vi "显示UI.vi"() -> ()   [LabVIEW 2016, in "国弘多参数.lvlib"]
uses:
  <vilib>/Utility/miscctls.llb/LVPointTypeDef.ctl
  <vilib>/Utility/config.llb/NI_LVConfig.lvlib
panel:
  in  "周期设置":bool
  out "运行状态":u16(ring) items=["空闲", "水样测试", "标样核查"]
  in  "叶绿素a校准":bool
  in  "停止":bool
  in  "标样核查":bool
  in  "水样测试":bool
  in  "open MB":bool
  in  "设置":bool
  in  "水温校准":bool
  in  "浊度校准":bool
  in  "溶解氧校准":bool
  in  "电导率校准":bool
  in  "pH校准":bool
  in  "探头校正返回":bool
  in  "探头校正":bool
  in  "浊度参数查询":bool
  in  "溶解氧参数查询":bool
  in  "电导率参数查询":bool
  in  "pH参数查询":bool
  out "检测值":T1
  in  "返回":bool
  in  "参数查询":bool
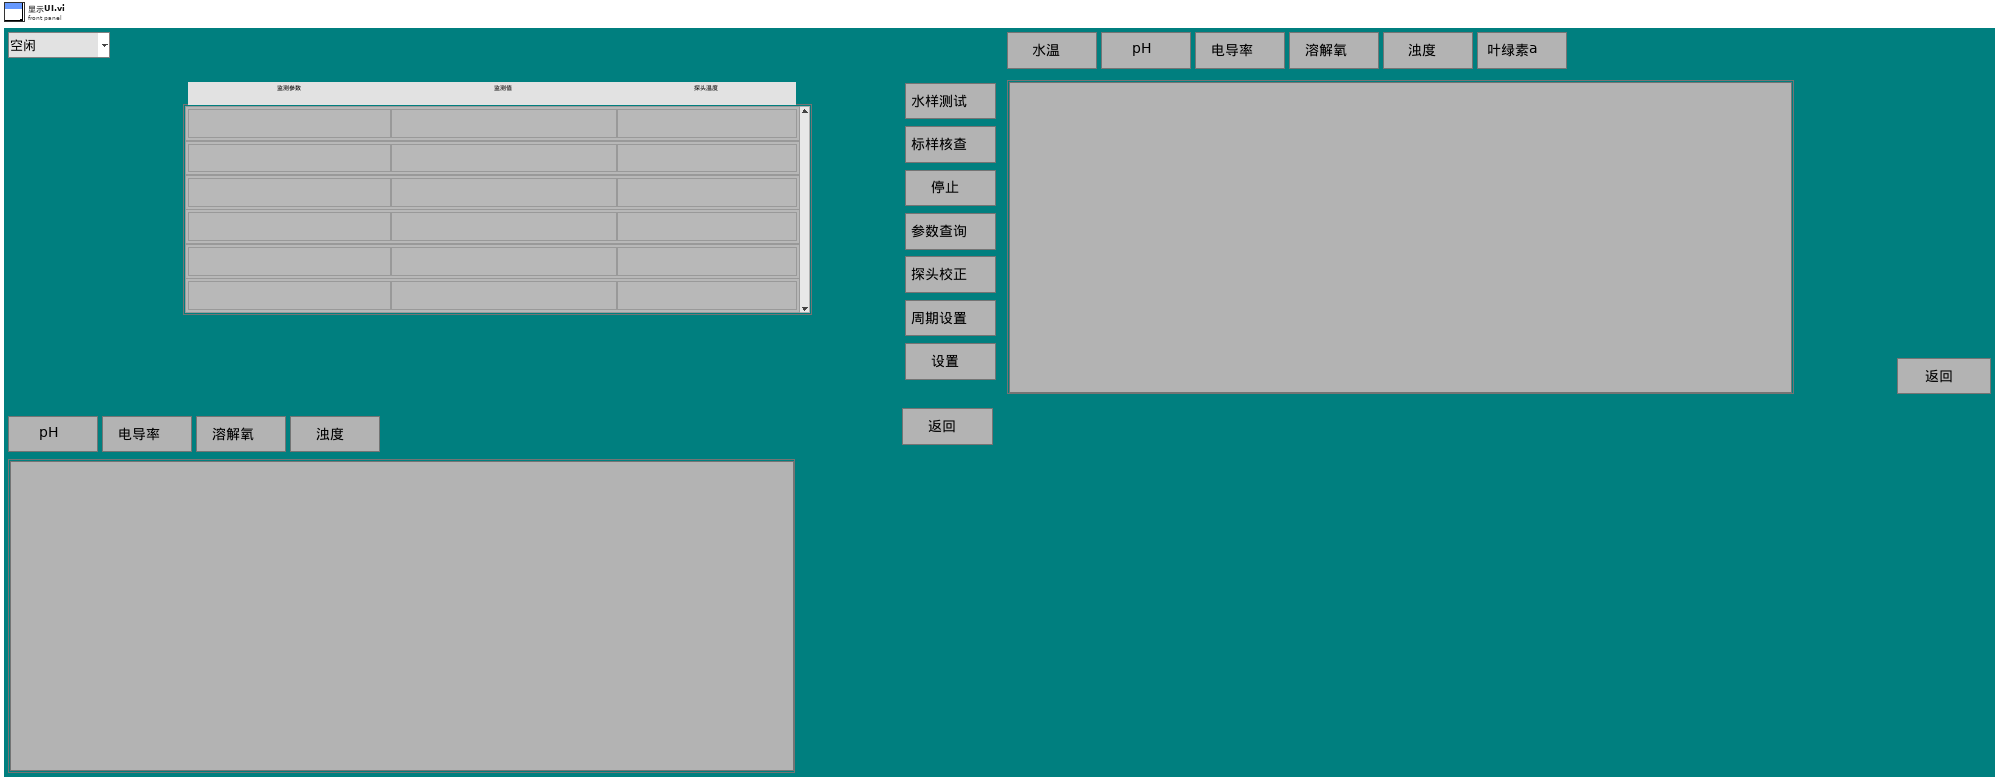
[diagram p1: front panel]
types:
  T1 = typedef "国弘多参数.lvlib/检测值.ctl" = cluster{"监测参数1":string, "浓度1":string, "探头温度1":string}[]
  T2 = typedef "LVPointTypeDef.ctl" = cluster{"Horizontal":i16, "Vertical":i16}
  T3 = cluster{"电极状态标志":u16, "电极型号标志":u16, "溶解氧测量值":sgl, "温度测量值":sgl, "溶解氧饱和度值":sgl, "盐度补偿值":sgl, "大气压补偿值":sgl, "溶解氧偏移修正值":sgl, "温度偏移修正值":sgl, "手动温度补偿值":sgl, "溶解氧电极零点":sgl, "溶解氧电极斜率":sgl, "第1点标准值记录":sgl, "第1点信号值记录":sgl, "第1点温度值记录":sgl, "第2点标准值记录":sgl, "第2点信号值记录":sgl, "第2点温度值记录":sgl, "命令滤波设定":u16, "温度模式":enum16{"ATC", "MTC"}, "生产批次":u16, "电极序号":u16, "串口地址":u16, "串口波特率":enum16{"9600", "19200", "115200"}, "串口校验位":enum16{"NONE", "ODD", "EVEN"}, "串口停止位":enum16{"1bit", "2bit"}, "第一点标准值":sgl, "第二点标准值":sgl}
  T4 = cluster{"电极状态标志":u16, "电极型号标志":u16, "酸碱度测量值":sgl, "温度测量值":sgl, "酸碱度信号值":sgl, "温度信号值":sgl, "酸碱度偏移修正值":sgl, "温度偏移修正值":sgl, "手动温度补偿值":sgl, "酸碱度电极零点":sgl, "酸碱度电极斜率":sgl, "第1点标准值记录":sgl, "第1点信号值记录":sgl, "第1点温度值记录":sgl, "第2点标准值记录":sgl, "第2点信号值记录":sgl, "第2点温度值记录":sgl, "命令滤波设定":u16, "温度模式":enum16{"ATC", "MTC"}, "生产批次":u16, "电极序号":u16, "串口地址":u16, "串口波特率":enum16{"9600", "19200", "115200"}, "串口校验位":enum16{"NONE", "ODD", "EVEN"}, "串口停止位":enum16{"1bit", "2bit"}, "第一点标准值":sgl, "第二点标准值":sgl}
  T5 = cluster{"电极状态标志":u16, "电极型号标志":u16, "浊度测量值":sgl, "温度测量值":sgl, "浊度信号值":sgl, "浊度偏移修正值":sgl, "温度偏移修正值":sgl, "手动温度补偿值":sgl, "浊度电极零点":sgl, "浊度电极斜率":sgl, "第1点标准值记录":sgl, "第1点信号值记录":sgl, "第1点温度值记录":sgl, "第2点标准值记录":sgl, "第2点信号值记录":sgl, "第2点温度值记录":sgl, "命令滤波设定":u16, "温度模式":enum16{"ATC", "MTC"}, "生产批次":u16, "电极序号":u16, "串口地址":u16, "串口波特率":enum16{"9600", "19200", "115200"}, "串口校验位":enum16{"NONE", "ODD", "EVEN"}, "串口停止位":enum16{"1bit", "2bit"}, "第一点标准值":sgl, "第二点标准值":sgl}
  T6 = cluster{"电极状态标志":u16, "电极型号标志":u16, "电导率测量值":sgl, "温度测量值":sgl, "电导率信号值":sgl, "温度信号值":sgl, "温度补偿系数":sgl, "电导率偏移修正值":sgl, "温度偏移修正值":sgl, "手动温度补偿值":sgl, "电导率电极零点":sgl, "电导率电极斜率":sgl, "命令滤波设定":u16, "温度模式":enum16{"ATC", "MTC"}, "生产批次":u16, "电极序号":u16, "串口地址":u16, "串口波特率":enum16{"9600", "19200", "115200"}, "串口校验位":enum16{"NONE", "ODD", "EVEN"}, "串口停止位":enum16{"1bit", "2bit"}, "第一点标准值":sgl, "第二点标准值":sgl}
  T7 = cluster{"监测参数1":string, "浓度1":string, "探头温度1":string}[]
  T8 = cluster{"CH":u16, "监测值":dbl, "监测信号值":dbl, "温度偏移修正值":sgl}
  T9 = typedef "NI_LVConfig.lvlib/Config Data RefNum.ctl" = refnum<k1>
  T10 = enum32{"Bad", "Idle", "Run top level", "Running"}
  T11 = cluster{"baud rate (bps)":u32, "stop bits":u16, "parity":u16, "flow control":u16, "timeout":u32, "retries":i32}
  T12 = enum32{"Invalid", "Standard", "Closed", "Hidden", "Minimized", "Maximized"}
  T13 = cluster{"数据保存间隔":dbl, "水温标样值":dbl, "pH标样值":dbl, "溶解氧标样值":dbl, "电导率标样值":dbl, "浊度标样值":dbl}
  T14 = cluster{"Temp":bool, "pH":bool, "DO":bool, "Cond":bool, "Turb":bool, "叶绿素a启用":bool}
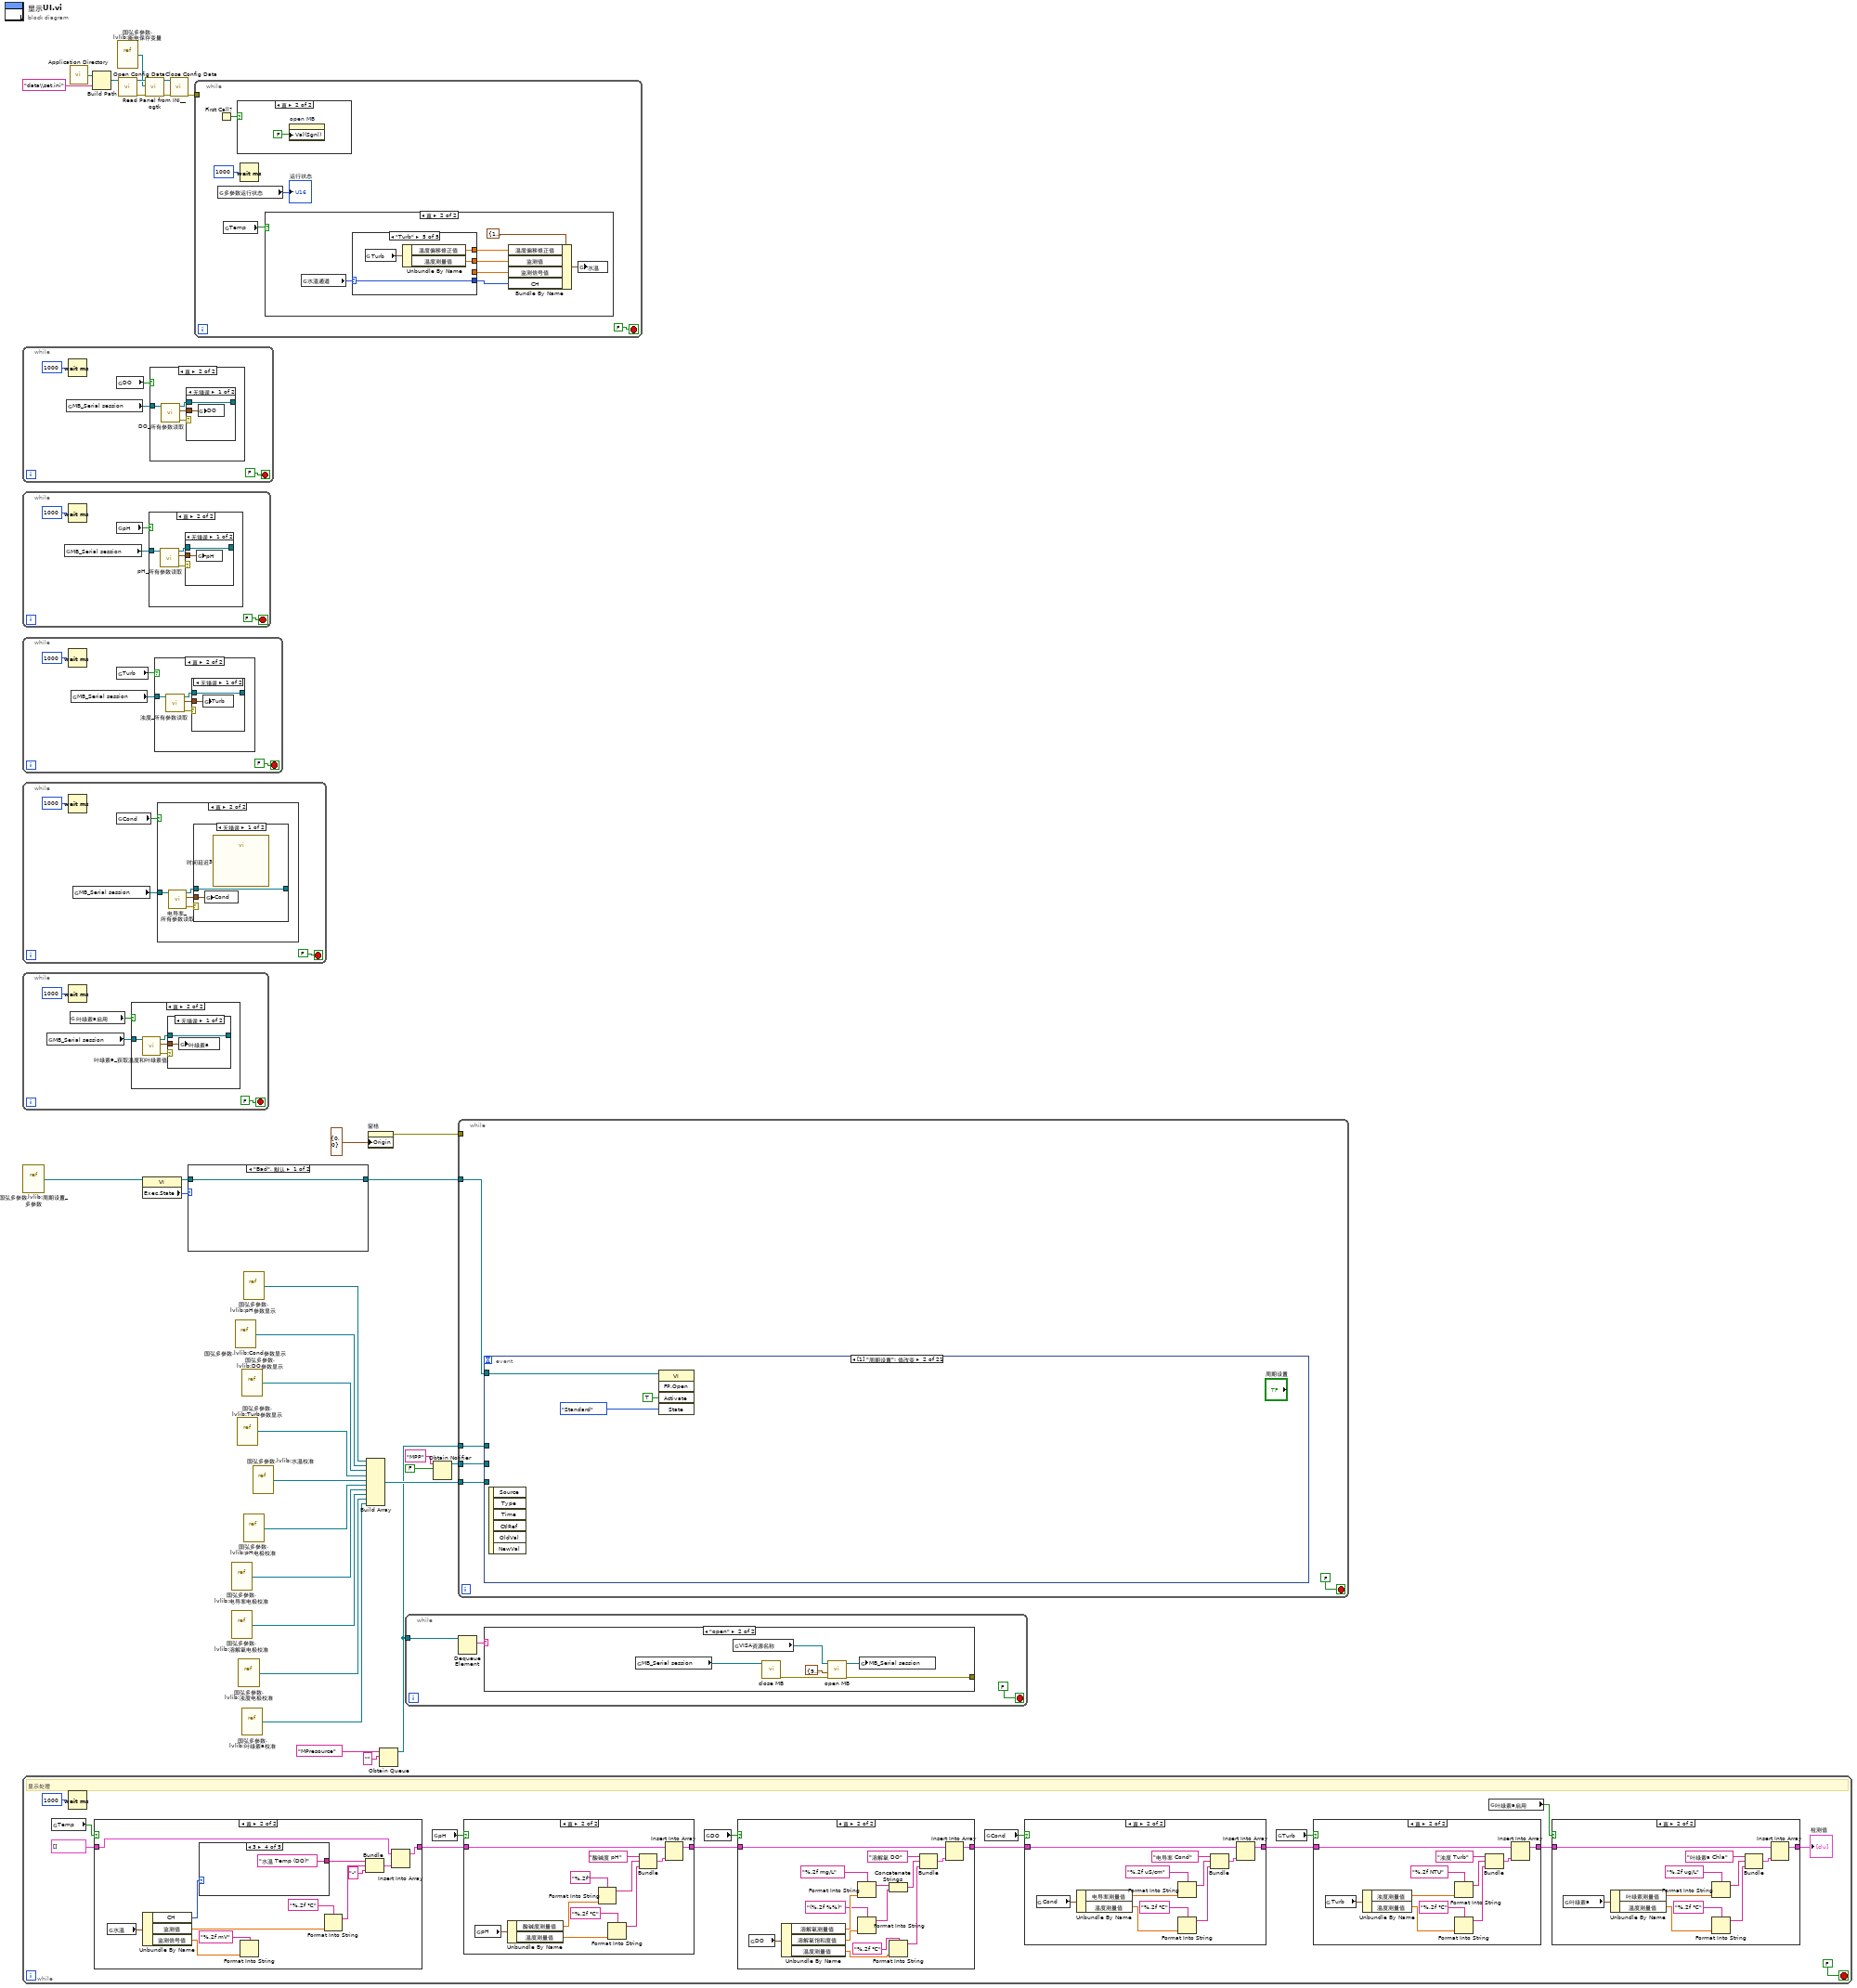
[diagram p0: block diagram]
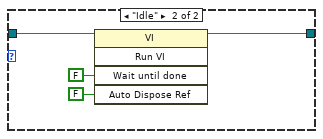
[diagram p2: hidden frame]
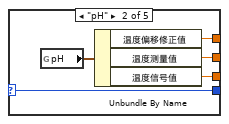
[diagram p16: hidden frame]
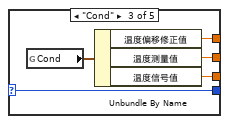
[diagram p17: hidden frame]
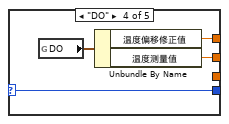
[diagram p18: hidden frame]
diagram:
  n1 = while {
    stop <- FALSE stop-if-true
    n2 = global read "过程全局变量.vi" "MB_Serial session"() -> (w33:refnum<class "MB_Master_Serial.lvclass">)
    n3 = Wait (ms)(milliseconds to wait=u32 1000 ("等待时间（毫秒）")) -> ()  [unwired: 1 out]
    n4 = global read "断电保存变量.vi" "DO"() -> (w34:bool)
    n5 = case shown="真" w34 {
      tunnel: w33 -> [_ w37]
      frame False {
      }
      frame True {
        n6 = call "DO_所有参数读取.vi"("MB_Serial session in"=w37) -> ("error out"=w39:errorcluster, "输出值"=w40:T3, "MB_Serial session out"=w38:refnum<class "MB_Master_Serial.lvclass">)  [unwired: 8 in]
        n7 = case shown="无错误" w39 {
          tunnel: w40 -> [w42 _]
          tunnel: w38 -> [w41 w43]
          tunnel: [w41 w43] -> _
          frame No Error {
            n8 = global write "过程全局变量.vi" "DO"(w42) -> ()
          }
          frame Error {
          }
        }
      }
    }
  }
  n9 = while {
    stop <- FALSE stop-if-true
    n10 = global read "过程全局变量.vi" "MB_Serial session"() -> (w45:refnum<class "MB_Master_Serial.lvclass">)
    n11 = Wait (ms)(milliseconds to wait=u32 1000 ("等待时间（毫秒）")) -> ()  [unwired: 1 out]
    n12 = global read "断电保存变量.vi" "pH"() -> (w46:bool)
    n13 = case shown="真" w46 {
      tunnel: w45 -> [_ w48]
      frame False {
      }
      frame True {
        n14 = call "pH_所有参数读取.vi"("MB_Serial session in"=w48) -> ("error out"=w50:errorcluster, "输出值"=w51:T4, "MB_Serial session out"=w49:refnum<class "MB_Master_Serial.lvclass">)  [unwired: 8 in]
        n15 = case shown="无错误" w50 {
          tunnel: w51 -> [w53 _]
          tunnel: w49 -> [w52 w54]
          tunnel: [w52 w54] -> _
          frame No Error {
            n16 = global write "过程全局变量.vi" "pH"(w53) -> ()
          }
          frame Error {
          }
        }
      }
    }
  }
  n17 = while {
    stop <- FALSE stop-if-true
    n18 = Wait (ms)(milliseconds to wait=u32 1000 ("等待时间（毫秒）")) -> ()  [unwired: 1 out]
    n19 = global read "过程全局变量.vi" "MB_Serial session"() -> (w56:refnum<class "MB_Master_Serial.lvclass">)
    n20 = global read "断电保存变量.vi" "Turb"() -> (w57:bool)
    n21 = case shown="真" w57 {
      tunnel: w56 -> [_ w59]
      frame False {
      }
      frame True {
        n22 = call "浊度_所有参数读取.vi"("MB_Serial session in"=w59) -> ("error out"=w61:errorcluster, "输出值"=w62:T5, "MB_Serial session out"=w60:refnum<class "MB_Master_Serial.lvclass">)  [unwired: 8 in]
        n23 = case shown="无错误" w61 {
          tunnel: w62 -> [w64 _]
          tunnel: w60 -> [w63 w65]
          tunnel: [w63 w65] -> _
          frame No Error {
            n24 = global write "过程全局变量.vi" "Turb"(w64) -> ()
          }
          frame Error {
          }
        }
      }
    }
  }
  n25 = while {
    stop <- FALSE stop-if-true
    n26 = Wait (ms)(milliseconds to wait=u32 1000 ("等待时间（毫秒）")) -> ()  [unwired: 1 out]
    n27 = global read "过程全局变量.vi" "MB_Serial session"() -> (w67:refnum<class "MB_Master_Serial.lvclass">)
    n28 = global read "断电保存变量.vi" "Cond"() -> (w68:bool)
    n29 = case shown="真" w68 {
      tunnel: w67 -> [_ w70]
      frame False {
      }
      frame True {
        n30 = call "电导率_所有参数读取.vi"("MB_Serial session in"=w70) -> ("error out"=w72:errorcluster, "输出值"=w73:T6, "MB_Serial session out"=w71:refnum<class "MB_Master_Serial.lvclass">)  [unwired: 8 in]
        n31 = case shown="无错误" w72 {
          tunnel: w73 -> [w75 _]
          tunnel: [w74 w76] -> _
          tunnel: w71 -> [w74 w76]
          frame No Error {
            n32 = global write "过程全局变量.vi" "Cond"(w75) -> ()
            n33 = call "时间延迟3"() -> ()  [unwired: 11 in, 1 out]
          }
          frame Error {
          }
        }
      }
    }
  }
  n34 = while {
    stop <- FALSE stop-if-true
    n35 = global read "过程全局变量.vi" "MB_Serial session"() -> (w79:refnum<class "MB_Master_Serial.lvclass">)
    n36 = Wait (ms)(milliseconds to wait=u32 1000 ("等待时间（毫秒）")) -> ()  [unwired: 1 out]
    n37 = global read "断电保存变量.vi" "叶绿素a启用"() -> (w78:bool)
    n38 = case shown="真" w78 {
      tunnel: w79 -> [_ w81]
      frame False {
      }
      frame True {
        n39 = call "叶绿素a_获取温度和叶绿素值.vi"("MB_Serial session in"=w81) -> ("error out"=w83:errorcluster, "输出值"=w84:cluster{"温度测量值":sgl, "叶绿素测量值":sgl, "错误标志":u16}, "MB_Serial session out"=w82:refnum<class "MB_Master_Serial.lvclass">)  [unwired: 8 in]
        n40 = case shown="无错误" w83 {
          tunnel: w84 -> [w86 _]
          tunnel: w82 -> [w85 w87]
          tunnel: [w85 w87] -> _
          frame No Error {
            n41 = global write "过程全局变量.vi" "叶绿素a"(w86) -> ()
          }
          frame Error {
          }
        }
      }
    }
  }
  n42 = vi-ref "国弘多参数.lvlib:周期设置_多参数.vi"() -> (w4:refnum<vi>)
  n43 = while {
    stop <- FALSE stop-if-true
    # "显示处理"
    n44 = global read "断电保存变量.vi" "Temp"() -> (w100:bool)
    n45 = Wait (ms)(milliseconds to wait=u32 1000 ("等待时间（毫秒）")) -> ()  [unwired: 1 out]
    n46 = case shown="真" w100 {
      tunnel: [w167 w168] -> w97
      tunnel: T7 [] ("数组") -> [w167 w169]
      frame False {
      }
      frame True {
        n47 = global read "过程全局变量.vi" "水温"() -> (w179:T8)
        n48 = Unbundle By Name(w179) -> ("CH"=w174:u16, "监测值"=w177:dbl, "监测信号值"=w175:dbl)
        n49 = case shown="3" w174 {
          tunnel: ["水温 Temp" ("监测参数1") "水温 Temp (pH)" ("监测参数1") "水温 Temp (Cond)" ("监测参数1") "水温 Temp (DO)" ("监测参数1") "水温 Temp (Turb)" ("监测参数1")] -> w173
          frame 0, Default {
          }
          frame 1 {
          }
          frame 2 {
          }
          frame 3 {
          }
          frame 4 {
          }
        }
        n50 = Format Into String(format string="%.2f mV" ("格式字符串"), w175) -> ()  [unwired: 2 in, 2 out]
        n51 = Format Into String(format string="%.2f ℃" ("格式字符串"), w177) -> (resulting string=w172:string)  [unwired: 2 in, 1 out]
        n52 = Bundle("监测参数1"=w173, w172, "探头温度1"="-") -> (w170:cluster{"监测参数1":string, string, "探头温度1":string})  [unwired: 1 in]
        n53 = Insert Into Array(array=w169, new element=w170) -> (w168:T7)  [unwired: 1 in]
      }
    }
    n54 = global read "断电保存变量.vi" "pH"() -> (w98:bool)
    n55 = case shown="真" w98 {
      tunnel: [w155 w156] -> w95
      tunnel: w97 -> [w155 w158]
      frame False {
      }
      frame True {
        n56 = global read "过程全局变量.vi" "pH"() -> (w166:T4)
        n57 = Unbundle By Name(w166) -> ("酸碱度测量值"=w165:sgl, "温度测量值"=w163:sgl)
        n58 = Format Into String(format string="%.2f" ("格式字符串"), w165) -> (resulting string=w159:string)  [unwired: 2 in, 1 out]
        n59 = Format Into String(format string="%.2f ℃" ("格式字符串"), w163) -> (resulting string=w161:string)  [unwired: 2 in, 1 out]
        n60 = Bundle("监测参数2"="酸碱度 pH", w159, w161) -> (w157:cluster{"监测参数2":string, string, string})  [unwired: 1 in]
        n61 = Insert Into Array(array=w158, new element=w157) -> (w156:T7)  [unwired: 1 in]
      }
    }
    n62 = global read "断电保存变量.vi" "DO"() -> (w96:bool)
    n63 = case shown="真" w96 {
      tunnel: [w139 w140] -> w92
      tunnel: w95 -> [w139 w141]
      frame False {
      }
      frame True {
        n64 = global read "过程全局变量.vi" "DO"() -> (w150:T3)
        n65 = Unbundle By Name(w150) -> ("溶解氧测量值"=w151:sgl, "溶解氧饱和度值"=w148:sgl, "温度测量值"=w153:sgl)
        n66 = Format Into String(format string="%.2f mg/L" ("格式字符串"), w151) -> (resulting string=w147:string)  [unwired: 2 in, 1 out]
        n67 = Format Into String(format string="(%.2f %%)" ("格式字符串"), w148) -> (resulting string=w146:string)  [unwired: 2 in, 1 out]
        n68 = Concatenate Strings(w147, w146) -> (w145:string)
        n69 = Format Into String(format string="%.2f ℃" ("格式字符串"), w153) -> (resulting string=w143:string)  [unwired: 2 in, 1 out]
        n70 = Bundle("监测参数2"="溶解氧 DO", w145, w143) -> (w142:cluster{"监测参数2":string, string, string})  [unwired: 1 in]
        n71 = Insert Into Array(array=w141, new element=w142) -> (w140:T7)  [unwired: 1 in]
      }
    }
    n72 = global read "断电保存变量.vi" "Cond"() -> (w94:bool)
    n73 = case shown="真" w94 {
      tunnel: w92 -> [w127 w130]
      tunnel: [w127 w128] -> w91
      frame False {
      }
      frame True {
        n74 = global read "过程全局变量.vi" "Cond"() -> (w138:T6)
        n75 = Unbundle By Name(w138) -> ("电导率测量值"=w137:sgl, "温度测量值"=w135:sgl)
        n76 = Format Into String(format string="%.2f uS/cm" ("格式字符串"), w137) -> (resulting string=w131:string)  [unwired: 2 in, 1 out]
        n77 = Format Into String(format string="%.2f ℃" ("格式字符串"), w135) -> (resulting string=w132:string)  [unwired: 2 in, 1 out]
        n78 = Bundle("监测参数2"="电导率 Cond", w131, w132) -> (w129:cluster{"监测参数2":string, string, string})  [unwired: 1 in]
        n79 = Insert Into Array(array=w130, new element=w129) -> (w128:T7)  [unwired: 1 in]
      }
    }
    n80 = global read "断电保存变量.vi" "Turb"() -> (w93:bool)
    n81 = case shown="真" w93 {
      tunnel: w91 -> [w115 w118]
      tunnel: [w115 w116] -> w90
      frame False {
      }
      frame True {
        n82 = global read "过程全局变量.vi" "Turb"() -> (w122:T5)
        n83 = Unbundle By Name(w122) -> ("浊度测量值"=w123:sgl, "温度测量值"=w125:sgl)
        n84 = Format Into String(format string="%.2f NTU" ("格式字符串"), w123) -> (resulting string=w120:string)  [unwired: 2 in, 1 out]
        n85 = Format Into String(format string="%.2f ℃" ("格式字符串"), w125) -> (resulting string=w121:string)  [unwired: 2 in, 1 out]
        n86 = Bundle("监测参数2"="浊度 Turb", w120, w121) -> (w117:cluster{"监测参数2":string, string, string})  [unwired: 1 in]
        n87 = Insert Into Array(array=w118, new element=w117) -> (w116:T7)  [unwired: 1 in]
      }
    }
    n88 = global read "断电保存变量.vi" "叶绿素a启用"() -> (w88:bool)
    n89 = case shown="真" w88 {
      tunnel: w90 -> [w103 w106]
      tunnel: [w103 w104] -> w89
      frame False {
      }
      frame True {
        n90 = global read "过程全局变量.vi" "叶绿素a"() -> (w110:cluster{"温度测量值":sgl, "叶绿素测量值":sgl, "错误标志":u16})
        n91 = Unbundle By Name(w110) -> ("叶绿素测量值"=w111:sgl, "温度测量值"=w113:sgl)
        n92 = Format Into String(format string="%.2f ug/L" ("格式字符串"), w111) -> (resulting string=w108:string)  [unwired: 2 in, 1 out]
        n93 = Format Into String(format string="%.2f ℃" ("格式字符串"), w113) -> (resulting string=w109:string)  [unwired: 2 in, 1 out]
        n94 = Bundle("监测参数2"="叶绿素a Chla", w108, w109) -> (w105:cluster{"监测参数2":string, string, string})  [unwired: 1 in]
        n95 = Insert Into Array(array=w106, new element=w105) -> (w104:T7)  [unwired: 1 in]
      }
    }
    "检测值" <- w89
  }
  n96 = call <vilib>:"Application Directory.vi"() -> ("Application Directory"=w16:path)
  n97 = Build Path(base path=w16, name or relative path="data\\set.ini" ("名称或相对路径")) -> (appended path=w15:path)
  n98 = vi-ref "国弘多参数.lvlib:断电保存变量.vi"() -> (w13:refnum<vi>)
  n99 = call <vilib>:"Open Config Data.vi"("configuration file path"=w15) -> ("error out"=w19:errorcluster, "refnum"=w20:T9)  [unwired: 8 in, 1 out]
  n100 = property class="VI"(reference=w4) -> (reference out=w2:refnum<vi>, "Exec.State"=w3:T10)  [unwired: 1 in, 1 out]
  n101 = call <userlib>:"Read Panel from INI__ogtk.vi"("error in (no error)"=w19, "VI ref"=w13, "refnum"=w20) -> ("error out"=w17:errorcluster, "refnum out"=w18:T9)  [unwired: 7 in]
  n102 = call <vilib>:"Close Config Data.vi"("error in (no error)"=w17, "refnum"=w18) -> ("error out"=w12:errorcluster)  [unwired: 8 in, 1 out]
  n103 = case shown="\"Bad\", 默认" w3 {
    tunnel: w2 -> [w185 w189]
    tunnel: [w185 w186] -> w1
    frame "Bad", Default {
    }
    frame "Idle" {
      n104 = invoke class="VI" method="Run VI"(reference=w189, "Wait until done"=FALSE ("结束前等待"), "Auto Dispose Ref"=FALSE ("自动销毁引用")) -> (reference out=w186:refnum<vi>)  [unwired: 2 in, 4 out]
    }
  }
  n105 = while {
    tunnel: w12 -> [_]
    stop <- FALSE stop-if-true
    n106 = First Call?() -> (First Call?: T/F=w192:bool)
    n107 = global read "过程全局变量.vi" "多参数运行状态"() -> (→"运行状态":u16)
    n108 = global read "断电保存变量.vi" "Temp"() -> (w191:bool)
    n109 = case shown="真" w192 {
      frame False {
      }
      frame True {
        n110 = property on="open MB" class="Bool (严格)"("Val(Sgnl)"=FALSE ("值(信号)")) -> ()  [unwired: 2 in, 2 out]
      }
    }
    n111 = Wait (ms)(milliseconds to wait=u32 1000 ("等待时间（毫秒）")) -> ()  [unwired: 1 out]
    n112 = case shown="真" w191 {
      frame False {
      }
      frame True {
        n113 = global read "断电保存变量.vi" "水温通道"() -> (w201:enum16{"NULL", "pH", "Cond", "DO", "Turb"})
        n114 = case shown="\"Turb\"" w201 {
          selector: w201 -> [w202 w207 w212 w216 w220]
          tunnel: [w202 w207 w212 w216 w220] -> w200
          tunnel: [_ w205 w210 w214 w218] -> w199
          tunnel: [_ w204 w209 _ _] -> w198
          tunnel: [_ w203 w208 w213 w217] -> w195
          frame "NULL", Default {
          }
          frame "pH" {
            n115 = global read "过程全局变量.vi" "pH"() -> (w206:T4)
            n116 = Unbundle By Name(w206) -> ("温度偏移修正值"=w203:sgl, "温度测量值"=w205:sgl, "温度信号值"=w204:sgl)
          }
          frame "Cond" {
            n117 = global read "过程全局变量.vi" "Cond"() -> (w211:T6)
            n118 = Unbundle By Name(w211) -> ("温度偏移修正值"=w208:sgl, "温度测量值"=w210:sgl, "温度信号值"=w209:sgl)
          }
          frame "DO" {
            n119 = global read "过程全局变量.vi" "DO"() -> (w215:T3)
            n120 = Unbundle By Name(w215) -> ("温度偏移修正值"=w213:sgl, "温度测量值"=w214:sgl)
          }
          frame "Turb" {
            n121 = global read "过程全局变量.vi" "Turb"() -> (w219:T5)
            n122 = Unbundle By Name(w219) -> ("温度偏移修正值"=w217:sgl, "温度测量值"=w218:sgl)
          }
        }
        n123 = Bundle By Name(cluster=T8 {"CH"=1, "监测值"=0.0, "监测信号值"=0.0, "温度偏移修正值"=0.0} ("水温"), "温度偏移修正值"=w195, "监测值"=w199, "监测信号值"=w198, "CH"=w200) -> (w197:T8)
        n124 = global write "过程全局变量.vi" "水温"(w197) -> ()
      }
    }
  }
  n125 = vi-ref "国弘多参数.lvlib:电导率电极校准.vi"() -> (w23:refnum<vi>)
  n126 = vi-ref "国弘多参数.lvlib:溶解氧电极校准.vi"() -> (w22:refnum<vi>)
  n127 = vi-ref "国弘多参数.lvlib:Cond参数显示.vi"() -> (w29:refnum<vi>)
  n128 = vi-ref "国弘多参数.lvlib:Turb参数显示.vi"() -> (w27:refnum<vi>)
  n129 = vi-ref "国弘多参数.lvlib:浊度电极校准.vi"() -> (w21:refnum<vi>)
  n130 = vi-ref "国弘多参数.lvlib:DO参数显示.vi"() -> (w28:refnum<vi>)
  n131 = vi-ref "国弘多参数.lvlib:叶绿素a校准.vi"() -> (w11:refnum<vi>)
  n132 = vi-ref "国弘多参数.lvlib:pH参数显示.vi"() -> (w30:refnum<vi>)
  n133 = vi-ref "国弘多参数.lvlib:pH电极校准.vi"() -> (w24:refnum<vi>)
  n134 = vi-ref "国弘多参数.lvlib:水温校准.vi"() -> (w25:refnum<vi>)
  n135 = Build Array(w30, w29, w28, w27, w25, w24, w23, w22, w21, w11) -> (w26:refnum<vi>[])
  n136 = property on="窗格" class="Pane"("Origin"=T2 {"Horizontal"=0, "Vertical"=0} ("原点")) -> (error out=w32:errorcluster)  [unwired: 2 in, 1 out]
  n137 = Obtain Queue(name (unnamed)="MPresource" ("名称（未命名）"), element data type="" ("名称（未命名）")) -> (queue out=w5:refnum<queue>)  [unwired: 3 in, 2 out]
  n138 = while {
    tunnel: w5 -> [w223]
    stop <- FALSE stop-if-true
    n139 = Dequeue Element(queue=w223) -> (element=w222:string)  [unwired: 2 in, 3 out]
    n140 = case shown="\"open\"" w222 {
      tunnel: [_ w225] -> _
      frame "假", Default {
      }
      frame "open" {
        n141 = global read "过程全局变量.vi" "MB_Serial session"() -> (w230:refnum<class "MB_Master_Serial.lvclass">)
        n142 = global read "断电保存变量.vi" "VISA资源名称"() -> (w227:refnum<visa-resource-name>)
        n143 = call "close MB.vi"("MB_Serial session"=w230) -> ("error out"=w229:errorcluster)  [unwired: 10 in]
        n144 = call "open MB.vi"("error in (no error)"=w229, "Serial Config"=T11 {"baud rate (bps)"=9600, "stop bits"=10, "parity"=0, "flow control"=0, "timeout"=1000, "retries"=1}, "VISA资源名称"=w227) -> ("error out"=w225:errorcluster, "MB_Serial session"=w228:refnum<class "MB_Master_Serial.lvclass">)  [unwired: 7 in]
        n145 = global write "过程全局变量.vi" "MB_Serial session"(w228) -> ()
      }
    }
  }
  n146 = Obtain Notifier(name (unnamed)="MPP" ("名称（未命名）"), notification data type=FALSE) -> (notifier out=w8:refnum<notifier>)  [unwired: 2 in, 2 out]
  n147 = while {
    tunnel: w32 -> [_]
    tunnel: w26 -> [w234]
    tunnel: w8 -> [w233]
    tunnel: w5 -> [w232]
    tunnel: w1 -> [w231]
    stop <- FALSE stop-if-true
    n148 = event shown="[1] \"周期设置\": 值改变" {
      selector: _ -> [_ _ _ _ _ _ _ _ _ _ _ _ _ _ _ _ _ _ _ _ _]
      dyn-events: _ -> [_ _ _ _ _ _ _ _ _ _ _ _ _ _ _ _ _ _ _ _ _]
      timeout: _ -> [_ _ _ _ _ _ _ _ _ _ _ _ _ _ _ _ _ _ _ _ _]
      tunnel: w234 -> [_ _ _ _ _ _ _ w297 w310 w322 w330 w342 w354 w366 w378 w390 w402 w414 w426 w438 w450]
      tunnel: w233 -> [_ _ _ _ w270 _ _ _ _ _ _ _ _ _ _ _ _ _ _ _ _]
      tunnel: w232 -> [_ _ _ _ _ w273 _ _ _ _ _ _ _ _ _ _ _ _ _ _ _]
      tunnel: w231 -> [_ w238 _ _ _ _ _ _ _ _ _ _ _ _ _ _ _ _ _ _ _]
      event Timeout {
        n149 = event-data() -> ()  [unwired: 1 in, 3 out]
      }
      event "周期设置": Value Change {
        n150 = event-data() -> ()  [unwired: 1 in, 6 out]
        n151 = invoke class="VI" method="FP.Open"(reference=w238, "Activate"=TRUE ("激活？"), "State"=T12."Standard" ("状态")) -> ()  [unwired: 2 in, 5 out]
      }
      event "水样测试": Value Change {
        n152 = event-data() -> ()  [unwired: 1 in, 6 out]
        n153 = call "水样测试配置.vi"() -> ("确认输出"=w240:bool, "水样测定时间输出"=w239:dbl)  [unwired: 10 in]
        n154 = case shown="真" w240 {
          tunnel: w239 -> [_ w243]
          frame False {
          }
          frame True {
            n155 = vi-ref "国弘多参数.lvlib:水样测试.vi"() -> (w244:refnum<vi>)
            n156 = property class="VI"(reference=w244) -> ("Name"=w248:string, "Exec.State"=w246:T10)  [unwired: 1 in, 2 out]
            n157 = Open VI Reference(type specifier VI Refnum (for type only)=refnum<vi> refnum, vi path=w248, options=128 ("选项")) -> (vi reference=w249:refnum<vi>)  [unwired: 3 in, 1 out]
            n158 = case shown="\"Idle\"" w246 {
              tunnel: [w250 w254] -> w245
              tunnel: w249 -> [w250 w253]
              tunnel: w243 -> [_ w252]
              tunnel: "hd" ("数据标记表") -> [_ w251]
              frame "Bad", Default {
              }
              frame "Idle" {
                n159 = call-by-ref "开始异步调用"(reference=w253, "数据标记表"=w251, "水样测试时间"=w252) -> (reference out=w254:refnum<vi>)  [unwired: 11 in, 1 out]
              }
            }
            n160 = Close Reference(reference=w245) -> ()  [unwired: 1 in, 1 out]
          }
        }
      }
      event "标样核查": Value Change {
        n161 = event-data() -> ()  [unwired: 1 in, 6 out]
        n162 = call "标样核查配置.vi"() -> ("确认输出"=w256:bool, "标样核查配置"=w255:T13)  [unwired: 10 in]
        n163 = case shown="真" w256 {
          tunnel: w255 -> [_ w257]
          frame False {
          }
          frame True {
            n164 = vi-ref "国弘多参数.lvlib:标样核查.vi"() -> (w258:refnum<vi>)
            n165 = property class="VI"(reference=w258) -> ("Name"=w263:string, "Exec.State"=w260:T10)  [unwired: 1 in, 2 out]
            n166 = Open VI Reference(type specifier VI Refnum (for type only)=refnum<vi> refnum, vi path=w263, options=128 ("选项")) -> (vi reference=w264:refnum<vi>)  [unwired: 3 in, 1 out]
            n167 = case shown="\"Idle\"" w260 {
              tunnel: [w265 w268] -> w259
              tunnel: w264 -> [w265 w267]
              tunnel: w257 -> [_ w266]
              frame "Bad", Default {
              }
              frame "Idle" {
                n168 = call-by-ref "开始异步调用"(reference=w267, "标样核查配置"=w266) -> (reference out=w268:refnum<vi>)  [unwired: 12 in, 1 out]
              }
            }
            n169 = Close Reference(reference=w259) -> ()  [unwired: 1 in, 1 out]
          }
        }
      }
      event "停止": Value Change {
        n170 = event-data() -> ()  [unwired: 1 in, 6 out]
        n171 = Send Notification(notification=TRUE ("通知"), notifier=w270) -> ()  [unwired: 1 in, 2 out]
      }
      event "open MB": Value Change {
        n172 = event-data() -> ()  [unwired: 1 in, 6 out]
        n173 = Flush Queue(queue=w273) -> (queue out=w272:refnum<queue>)  [unwired: 1 in, 2 out]
        n174 = Enqueue Element(queue=w272, element="open" ("元素")) -> ()  [unwired: 2 in, 3 out]
      }
      event "设置": Value Change {
        n175 = event-data() -> ()  [unwired: 1 in, 6 out]
        n176 = flat-sequence {
          frame #0 {
            n177 = call "配置.vi"() -> ("启用参数"=w280:T14, "串口输出"=w281:refnum<visa-resource-name>)  [unwired: 10 in]
            n178 = global write "断电保存变量.vi" "VISA资源名称"(w281) -> ()
            n179 = Unbundle By Name(w280) -> ("Temp"=w275:bool, "pH"=w276:bool, "DO"=w277:bool, "Cond"=w278:bool, "Turb"=w279:bool, "叶绿素a启用"=w274:bool)
            n180 = global write "断电保存变量.vi" "pH"(w276) -> ()
            n181 = global write "断电保存变量.vi" "DO"(w277) -> ()
            n182 = global write "断电保存变量.vi" "Cond"(w278) -> ()
            n183 = global write "断电保存变量.vi" "Turb"(w279) -> ()
            n184 = global write "断电保存变量.vi" "Temp"(w275) -> ()
            n185 = global write "断电保存变量.vi" "叶绿素a启用"(w274) -> ()
          }
          frame #1 {
            n186 = call <vilib>:"Application Directory.vi"() -> ("Application Directory"=w291:path)
            n187 = Build Path(base path=w291, name or relative path="data\\set.ini" ("名称或相对路径")) -> (appended path=w290:path)
            n188 = call <vilib>:"Open Config Data.vi"("configuration file path"=w290) -> ("error out"=w294:errorcluster, "refnum"=w295:T9)  [unwired: 8 in, 1 out]
            n189 = vi-ref "国弘多参数.lvlib:断电保存变量.vi"() -> (w288:refnum<vi>)
            n190 = call <userlib>:"Write Panel to INI__ogtk.vi"("error in (no error)"=w294, "VI ref"=w288, "refnum"=w295) -> ("error out"=w292:errorcluster, "refnum out"=w293:T9)  [unwired: 7 in]
            n191 = call <vilib>:"Close Config Data.vi"("error in (no error)"=w292, "refnum"=w293) -> ("error out"=w284:errorcluster, "file path"=w285:path)  [unwired: 8 in]
            n192 = Open/Create/Replace File(file path (use dialog)=w285, error in=w284) -> (refnum out=w286:refnum<file>, error out=w287:errorcluster)  [unwired: 4 in, 1 out]
            n193 = Flush File(refnum=w286, error in=w287) -> (refnum out=w282:refnum<file>, error out=w283:errorcluster)
            n194 = Close File(refnum=w282, error in=w283) -> ()  [unwired: 2 out]
          }
          frame #2 {
            n195 = property on="open MB" class="Bool (严格)"("Val(Sgnl)"=FALSE ("值(信号)")) -> ()  [unwired: 2 in, 2 out]
          }
        }
      }
      event "探头校正返回": Value Change {
        n196 = event-data() -> ()  [unwired: 1 in, 6 out]
        n197 = disable-structure shown="禁用" {
          disable-tunnel: w297 -> [w299 _]
          frame Disabled {
            n198 = for {
              tunnel: w299 -> [w302] mode=indexing
              n199 = property class="VI"(reference=w302) -> (reference out=w300:refnum<vi>, "Exec.State"=w301:T10)  [unwired: 1 in, 1 out]
              n200 = case shown="\"Run top level\"" w301 {
                tunnel: w300 -> [_ _ w303 w304]
                frame "Bad", Default {
                }
                frame "Idle" {
                }
                frame "Run top level" {
                  n201 = invoke class="VI" method="Abort VI"(reference=w303) -> ()  [unwired: 2 in, 3 out]
                }
                frame "Running" {
                  n202 = invoke class="VI" method="Abort VI"(reference=w304) -> ()  [unwired: 2 in, 3 out]
                }
              }
            }
          }
          frame Enabled {
          }
        }
        n203 = property on="窗格" class="Pane"("Origin"=T2 {"Horizontal"=0, "Vertical"=0} ("原点")) -> ()  [unwired: 2 in, 2 out]
      }
      event "探头校正": Value Change {
        n204 = event-data() -> ()  [unwired: 1 in, 6 out]
        n205 = property on="窗格" class="Pane"("Origin"=T2 {"Horizontal"=1656, "Vertical"=0} ("原点")) -> ()  [unwired: 2 in, 2 out]
        n206 = Index Array(array=w310, index=4 ("索引")) -> (element=w311:refnum<vi>)
        n207 = property class="VI"(reference=w311) -> (reference out=w306:refnum<vi>, "Exec.State"=w305:T10)  [unwired: 1 in, 1 out]
        n208 = case shown="\"Bad\", 默认" w305 {
          tunnel: [w313 w315] -> w309
          tunnel: w306 -> [w313 w314]
          frame "Bad", Default {
          }
          frame "Idle" {
            n209 = invoke class="VI" method="Run VI"(reference=w314, "Wait until done"=FALSE ("结束前等待"), "Auto Dispose Ref"=FALSE ("自动销毁引用")) -> (reference out=w315:refnum<vi>)  [unwired: 2 in, 4 out]
          }
        }
        n210 = invoke on="探头校准子面板" class="SubPnl" method="Remove VI"() -> (error out=w308:errorcluster)  [unwired: 3 in, 2 out]
        n211 = invoke on="探头校准子面板" class="SubPnl" method="Insert VI"(error in=w308, "VI Ref"=w309) -> ()  [unwired: 2 in, 4 out]
      }
      event "参数查询": Value Change {
        n212 = event-data() -> ()  [unwired: 1 in, 6 out]
        n213 = property on="窗格" class="Pane"("Origin"=T2 {"Horizontal"=0, "Vertical"=628} ("原点")) -> ()  [unwired: 2 in, 2 out]
        n214 = Index Array(array=w322) -> (element=w323:refnum<vi>)  [unwired: 1 in]
        n215 = property class="VI"(reference=w323) -> (reference out=w319:refnum<vi>, "Exec.State"=w318:T10)  [unwired: 1 in, 1 out]
        n216 = case shown="\"Bad\", 默认" w318 {
          tunnel: [w325 w327] -> w321
          tunnel: w319 -> [w325 w326]
          frame "Bad", Default {
          }
          frame "Idle" {
            n217 = invoke class="VI" method="Run VI"(reference=w326, "Wait until done"=FALSE ("结束前等待"), "Auto Dispose Ref"=FALSE ("自动销毁引用")) -> (reference out=w327:refnum<vi>)  [unwired: 2 in, 4 out]
          }
        }
        n218 = invoke on="参数查询子面板" class="SubPnl" method="Remove VI"() -> (error out=w320:errorcluster)  [unwired: 3 in, 2 out]
        n219 = invoke on="参数查询子面板" class="SubPnl" method="Insert VI"(error in=w320, "VI Ref"=w321) -> ()  [unwired: 2 in, 4 out]
      }
      event "返回": Value Change {
        n220 = event-data() -> ()  [unwired: 1 in, 6 out]
        n221 = property on="窗格" class="Pane"("Origin"=T2 {"Horizontal"=0, "Vertical"=0} ("原点")) -> ()  [unwired: 2 in, 2 out]
        n222 = disable-structure shown="禁用" {
          disable-tunnel: w330 -> [w332 _]
          frame Disabled {
            n223 = for {
              tunnel: w332 -> [w335] mode=indexing
              n224 = property class="VI"(reference=w335) -> (reference out=w333:refnum<vi>, "Exec.State"=w334:T10)  [unwired: 1 in, 1 out]
              n225 = case shown="\"Run top level\"" w334 {
                tunnel: w333 -> [_ _ w336 w337]
                frame "Bad", Default {
                }
                frame "Idle" {
                }
                frame "Run top level" {
                  n226 = invoke class="VI" method="Abort VI"(reference=w336) -> ()  [unwired: 2 in, 3 out]
                }
                frame "Running" {
                  n227 = invoke class="VI" method="Abort VI"(reference=w337) -> ()  [unwired: 2 in, 3 out]
                }
              }
            }
          }
          frame Enabled {
          }
        }
      }
      event "pH参数查询": Value Change {
        n228 = event-data() -> ()  [unwired: 1 in, 6 out]
        n229 = Index Array(array=w342) -> (element=w343:refnum<vi>)  [unwired: 1 in]
        n230 = property class="VI"(reference=w343) -> (reference out=w339:refnum<vi>, "Exec.State"=w338:T10)  [unwired: 1 in, 1 out]
        n231 = case shown="\"Bad\", 默认" w338 {
          tunnel: [w344 w346] -> w341
          tunnel: w339 -> [w344 w345]
          frame "Bad", Default {
          }
          frame "Idle" {
            n232 = invoke class="VI" method="Run VI"(reference=w345, "Wait until done"=FALSE ("结束前等待"), "Auto Dispose Ref"=FALSE ("自动销毁引用")) -> (reference out=w346:refnum<vi>)  [unwired: 2 in, 4 out]
          }
        }
        n233 = invoke on="参数查询子面板" class="SubPnl" method="Remove VI"() -> (error out=w340:errorcluster)  [unwired: 3 in, 2 out]
        n234 = invoke on="参数查询子面板" class="SubPnl" method="Insert VI"(error in=w340, "VI Ref"=w341) -> ()  [unwired: 2 in, 4 out]
      }
      event "电导率参数查询": Value Change {
        n235 = event-data() -> ()  [unwired: 1 in, 6 out]
        n236 = Index Array(array=w354, index=1 ("索引")) -> (element=w355:refnum<vi>)
        n237 = property class="VI"(reference=w355) -> (reference out=w350:refnum<vi>, "Exec.State"=w349:T10)  [unwired: 1 in, 1 out]
        n238 = case shown="\"Bad\", 默认" w349 {
          tunnel: w350 -> [w356 w360]
          tunnel: [w356 w357] -> w352
          frame "Bad", Default {
          }
          frame "Idle" {
            n239 = invoke class="VI" method="Run VI"(reference=w360, "Wait until done"=FALSE ("结束前等待"), "Auto Dispose Ref"=FALSE ("自动销毁引用")) -> (reference out=w357:refnum<vi>)  [unwired: 2 in, 4 out]
          }
        }
        n240 = invoke on="参数查询子面板" class="SubPnl" method="Remove VI"() -> (error out=w351:errorcluster)  [unwired: 3 in, 2 out]
        n241 = invoke on="参数查询子面板" class="SubPnl" method="Insert VI"(error in=w351, "VI Ref"=w352) -> ()  [unwired: 2 in, 4 out]
      }
      event "溶解氧参数查询": Value Change {
        n242 = event-data() -> ()  [unwired: 1 in, 6 out]
        n243 = Index Array(array=w366, index=2 ("索引")) -> (element=w367:refnum<vi>)
        n244 = property class="VI"(reference=w367) -> (reference out=w362:refnum<vi>, "Exec.State"=w361:T10)  [unwired: 1 in, 1 out]
        n245 = case shown="\"Bad\", 默认" w361 {
          tunnel: [w368 w370] -> w364
          tunnel: w362 -> [w368 w369]
          frame "Bad", Default {
          }
          frame "Idle" {
            n246 = invoke class="VI" method="Run VI"(reference=w369, "Wait until done"=FALSE ("结束前等待"), "Auto Dispose Ref"=FALSE ("自动销毁引用")) -> (reference out=w370:refnum<vi>)  [unwired: 2 in, 4 out]
          }
        }
        n247 = invoke on="参数查询子面板" class="SubPnl" method="Remove VI"() -> (error out=w363:errorcluster)  [unwired: 3 in, 2 out]
        n248 = invoke on="参数查询子面板" class="SubPnl" method="Insert VI"(error in=w363, "VI Ref"=w364) -> ()  [unwired: 2 in, 4 out]
      }
      event "浊度参数查询": Value Change {
        n249 = event-data() -> ()  [unwired: 1 in, 6 out]
        n250 = Index Array(array=w378, index=3 ("索引")) -> (element=w379:refnum<vi>)
        n251 = property class="VI"(reference=w379) -> (reference out=w374:refnum<vi>, "Exec.State"=w373:T10)  [unwired: 1 in, 1 out]
        n252 = case shown="\"Bad\", 默认" w373 {
          tunnel: [w380 w382] -> w376
          tunnel: w374 -> [w380 w381]
          frame "Bad", Default {
          }
          frame "Idle" {
            n253 = invoke class="VI" method="Run VI"(reference=w381, "Wait until done"=FALSE ("结束前等待"), "Auto Dispose Ref"=FALSE ("自动销毁引用")) -> (reference out=w382:refnum<vi>)  [unwired: 2 in, 4 out]
          }
        }
        n254 = invoke on="参数查询子面板" class="SubPnl" method="Remove VI"() -> (error out=w375:errorcluster)  [unwired: 3 in, 2 out]
        n255 = invoke on="参数查询子面板" class="SubPnl" method="Insert VI"(error in=w375, "VI Ref"=w376) -> ()  [unwired: 2 in, 4 out]
      }
      event "水温校准": Value Change {
        n256 = event-data() -> ()  [unwired: 1 in, 6 out]
        n257 = Index Array(array=w390, index=4 ("索引")) -> (element=w391:refnum<vi>)
        n258 = property class="VI"(reference=w391) -> (reference out=w386:refnum<vi>, "Exec.State"=w385:T10)  [unwired: 1 in, 1 out]
        n259 = case shown="\"Bad\", 默认" w385 {
          tunnel: [w392 w394] -> w388
          tunnel: w386 -> [w392 w393]
          frame "Bad", Default {
          }
          frame "Idle" {
            n260 = invoke class="VI" method="Run VI"(reference=w393, "Wait until done"=FALSE ("结束前等待"), "Auto Dispose Ref"=FALSE ("自动销毁引用")) -> (reference out=w394:refnum<vi>)  [unwired: 2 in, 4 out]
          }
        }
        n261 = invoke on="探头校准子面板" class="SubPnl" method="Remove VI"() -> (error out=w387:errorcluster)  [unwired: 3 in, 2 out]
        n262 = invoke on="探头校准子面板" class="SubPnl" method="Insert VI"(error in=w387, "VI Ref"=w388) -> ()  [unwired: 2 in, 4 out]
      }
      event "pH校准": Value Change {
        n263 = event-data() -> ()  [unwired: 1 in, 6 out]
        n264 = Index Array(array=w402, index=5 ("索引")) -> (element=w403:refnum<vi>)
        n265 = property class="VI"(reference=w403) -> (reference out=w398:refnum<vi>, "Exec.State"=w397:T10)  [unwired: 1 in, 1 out]
        n266 = case shown="\"Bad\", 默认" w397 {
          tunnel: w398 -> [w404 w408]
          tunnel: [w404 w405] -> w400
          frame "Bad", Default {
          }
          frame "Idle" {
            n267 = invoke class="VI" method="Run VI"(reference=w408, "Wait until done"=FALSE ("结束前等待"), "Auto Dispose Ref"=FALSE ("自动销毁引用")) -> (reference out=w405:refnum<vi>)  [unwired: 2 in, 4 out]
          }
        }
        n268 = invoke on="探头校准子面板" class="SubPnl" method="Remove VI"() -> (error out=w399:errorcluster)  [unwired: 3 in, 2 out]
        n269 = invoke on="探头校准子面板" class="SubPnl" method="Insert VI"(error in=w399, "VI Ref"=w400) -> ()  [unwired: 2 in, 4 out]
      }
      event "电导率校准": Value Change {
        n270 = event-data() -> ()  [unwired: 1 in, 6 out]
        n271 = Index Array(array=w414, index=6 ("索引")) -> (element=w415:refnum<vi>)
        n272 = property class="VI"(reference=w415) -> (reference out=w410:refnum<vi>, "Exec.State"=w409:T10)  [unwired: 1 in, 1 out]
        n273 = case shown="\"Bad\", 默认" w409 {
          tunnel: [w416 w418] -> w412
          tunnel: w410 -> [w416 w417]
          frame "Bad", Default {
          }
          frame "Idle" {
            n274 = invoke class="VI" method="Run VI"(reference=w417, "Wait until done"=FALSE ("结束前等待"), "Auto Dispose Ref"=FALSE ("自动销毁引用")) -> (reference out=w418:refnum<vi>)  [unwired: 2 in, 4 out]
          }
        }
        n275 = invoke on="探头校准子面板" class="SubPnl" method="Remove VI"() -> (error out=w411:errorcluster)  [unwired: 3 in, 2 out]
        n276 = invoke on="探头校准子面板" class="SubPnl" method="Insert VI"(error in=w411, "VI Ref"=w412) -> ()  [unwired: 2 in, 4 out]
      }
      event "溶解氧校准": Value Change {
        n277 = event-data() -> ()  [unwired: 1 in, 6 out]
        n278 = Index Array(array=w426, index=7 ("索引")) -> (element=w427:refnum<vi>)
        n279 = property class="VI"(reference=w427) -> (reference out=w422:refnum<vi>, "Exec.State"=w421:T10)  [unwired: 1 in, 1 out]
        n280 = case shown="\"Bad\", 默认" w421 {
          tunnel: [w428 w430] -> w424
          tunnel: w422 -> [w428 w429]
          frame "Bad", Default {
          }
          frame "Idle" {
            n281 = invoke class="VI" method="Run VI"(reference=w429, "Wait until done"=FALSE ("结束前等待"), "Auto Dispose Ref"=FALSE ("自动销毁引用")) -> (reference out=w430:refnum<vi>)  [unwired: 2 in, 4 out]
          }
        }
        n282 = invoke on="探头校准子面板" class="SubPnl" method="Remove VI"() -> (error out=w423:errorcluster)  [unwired: 3 in, 2 out]
        n283 = invoke on="探头校准子面板" class="SubPnl" method="Insert VI"(error in=w423, "VI Ref"=w424) -> ()  [unwired: 2 in, 4 out]
      }
      event "浊度校准": Value Change {
        n284 = event-data() -> ()  [unwired: 1 in, 6 out]
        n285 = Index Array(array=w438, index=8 ("索引")) -> (element=w439:refnum<vi>)
        n286 = property class="VI"(reference=w439) -> (reference out=w434:refnum<vi>, "Exec.State"=w433:T10)  [unwired: 1 in, 1 out]
        n287 = case shown="\"Bad\", 默认" w433 {
          tunnel: [w440 w442] -> w436
          tunnel: w434 -> [w440 w441]
          frame "Bad", Default {
          }
          frame "Idle" {
            n288 = invoke class="VI" method="Run VI"(reference=w441, "Wait until done"=FALSE ("结束前等待"), "Auto Dispose Ref"=FALSE ("自动销毁引用")) -> (reference out=w442:refnum<vi>)  [unwired: 2 in, 4 out]
          }
        }
        n289 = invoke on="探头校准子面板" class="SubPnl" method="Remove VI"() -> (error out=w435:errorcluster)  [unwired: 3 in, 2 out]
        n290 = invoke on="探头校准子面板" class="SubPnl" method="Insert VI"(error in=w435, "VI Ref"=w436) -> ()  [unwired: 2 in, 4 out]
      }
      event "叶绿素a校准": Value Change {
        n291 = event-data() -> ()  [unwired: 1 in, 6 out]
        n292 = Index Array(array=w450, index=9 ("索引")) -> (element=w451:refnum<vi>)
        n293 = property class="VI"(reference=w451) -> (reference out=w446:refnum<vi>, "Exec.State"=w445:T10)  [unwired: 1 in, 1 out]
        n294 = case shown="\"Bad\", 默认" w445 {
          tunnel: [w452 w454] -> w448
          tunnel: w446 -> [w452 w453]
          frame "Bad", Default {
          }
          frame "Idle" {
            n295 = invoke class="VI" method="Run VI"(reference=w453, "Wait until done"=FALSE ("结束前等待"), "Auto Dispose Ref"=FALSE ("自动销毁引用")) -> (reference out=w454:refnum<vi>)  [unwired: 2 in, 4 out]
          }
        }
        n296 = invoke on="探头校准子面板" class="SubPnl" method="Remove VI"() -> (error out=w447:errorcluster)  [unwired: 3 in, 2 out]
        n297 = invoke on="探头校准子面板" class="SubPnl" method="Insert VI"(error in=w447, "VI Ref"=w448) -> ()  [unwired: 2 in, 4 out]
      }
    }
  }
